vi "DuelistTactic.vi"(9 "Game in":refnum<class "Game.lvclass">, 10 "Robot":refnum<class "Robot.lvclass">, 11 "DuelistTactic in":refnum<class "DuelistTactic.lvclass">) -> (2 "Robot out":refnum<class "Robot.lvclass">, 3 "DuelistTactic out":refnum<class "DuelistTactic.lvclass">)   [LabVIEW 2020, in "DuelistTactic.lvclass"]
uses:
  DuelistTactic.lvclass
  C:/Users/anton/Desktop/RoboIME/IC/SSL_AI/Tactic_class/Tactic.lvclass
  Robot_class/Robot.lvclass
  Game_class/Game.lvclass
  Robot_class/tactics.ctl
  Tactic_class/Tactic.lvclass/Tactic.ctl
  Robot_class/Robot.lvclass/Robot.ctl
  Tactic_class/Read Skillbook.vi
  Robot_class/Write tactic.vi
  Skillbook_class/Skillbook.lvclass
  DuelistSkill_class/DuelistSkill.lvclass
panel:
  out "x .or. y?":bool
  out "error out 2":errorcluster
  in  "error in (no error) 2":errorcluster
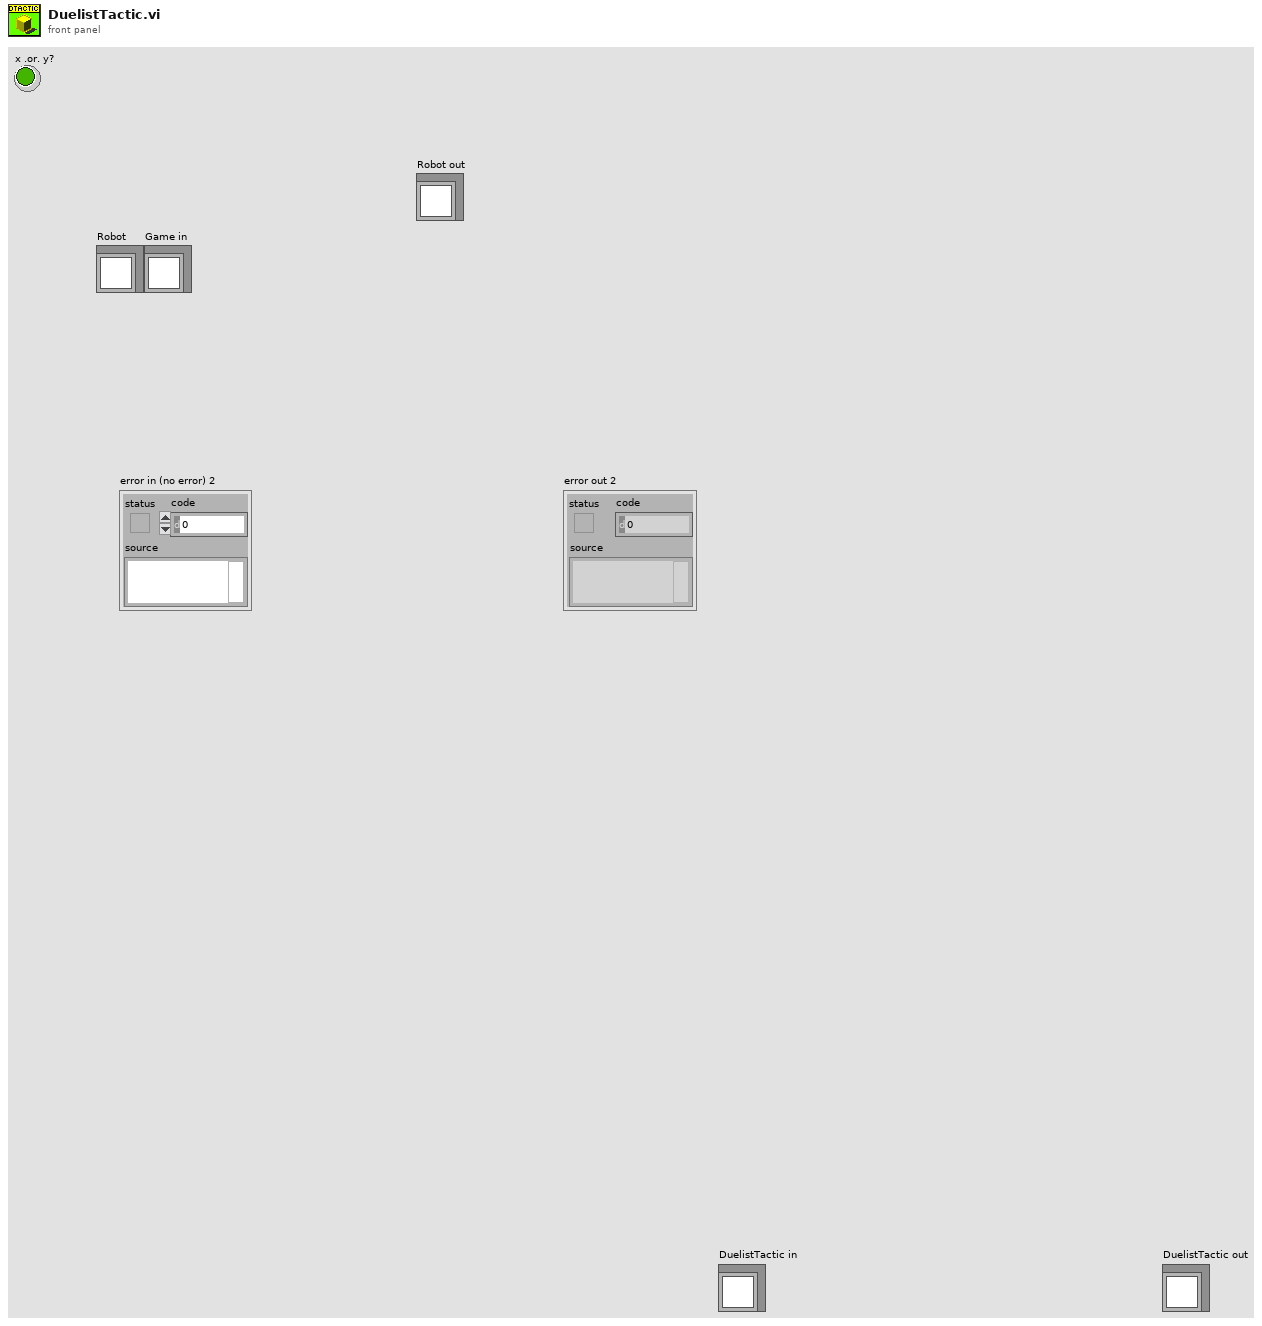
[diagram p1: front panel]
types:
  T1 = typedef "tactics.ctl" = enum16{"GoToBallPlacementPosition", "PlaceBall", "GoToBallPlacement", "5Robots", "BallPlacementEnemy", "ReceivePassInFuturePoint", "Roller", "PrepareRollToPassRollerGoTo", "PrepareRollToPassReceiverGoTo", "WaitRoll", "PositionToRoll", "PenaltyAttacker", "PassObserver", "PenaltyDefense", "TableReceiverTactic", "Test", "DefendGoal", "Marker", "FollowAttacker", "DefendArea", "Shoot", "AttackerAimGoal", "AttackerBallOutOfField", "AttackerBlock", "AttackerStop", "Duelist", "Halt", "ZigZag", "GoTo", "Timeout", "KickToBestRobot", "KickToPassReceiver", "PositionToReceivePass", "WaitPass"}
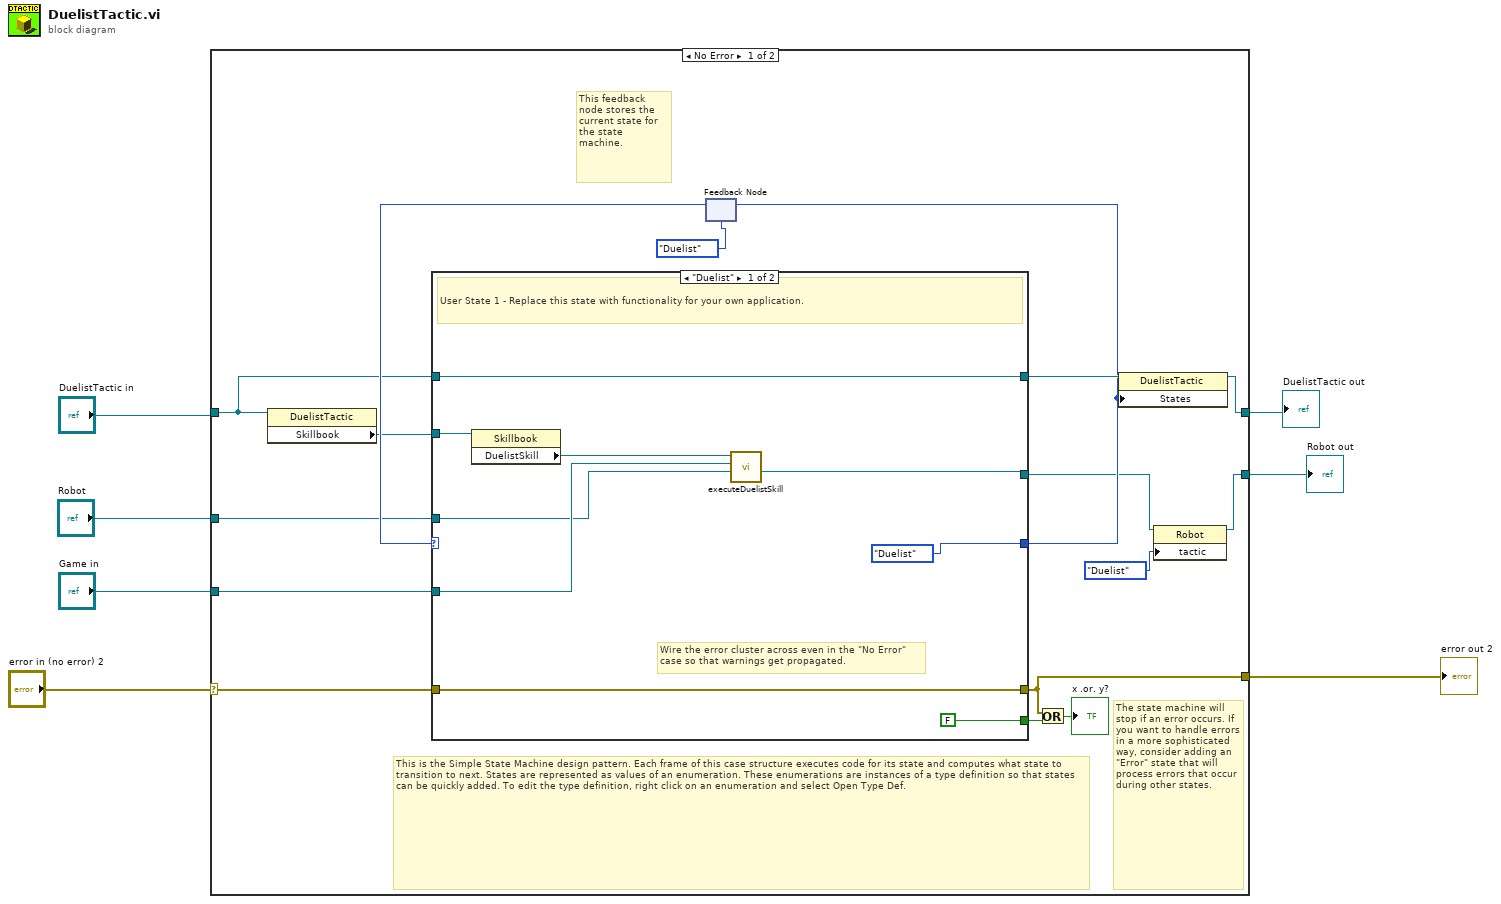
[diagram p0: block diagram]
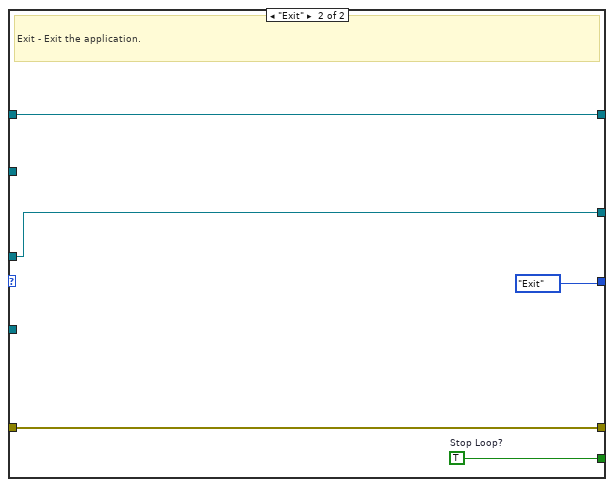
[diagram p2: hidden frame]
diagram:
  n1 = case shown="No Error" "error in (no error) 2" {
    selector: "error in (no error) 2" -> [w20 w40]
    tunnel: [w19 w40] -> w6
    tunnel: [w14 w39] -> w1
    tunnel: "DuelistTactic in" -> [w17 w39]
    tunnel: "Robot" -> [w18 w38]
    tunnel: [w8 w38] -> w4
    tunnel: "Game in" -> [w12 _]
    frame No Error {
      # "The state machine will stop if an error occurs. If you want to handle errors in a more sophisticated way, consider adding an \"Error\" state that will process errors that occur during other states."
      # "This feedback node stores the current state for the state machine."
      # "This is the Simple State Machine design pattern. Each frame of this case structure executes code for its state and computes what state to transition to next. States are represented as values of an enumeration. These enumerations are instances of a type definition so that states can be quickly added. To edit the type definition, right click on an enumeration and select Open Type Def."
      # "Wire the error cluster across even in the \"No Error\"\ncase so that warnings get propagated."
      n2 = property class="DuelistTactic"(reference=w17) -> ("Skillbook"=w16:refnum<class "Skillbook.lvclass">)  [unwired: 1 in, 2 out]
      n3 = feedback #1(enum16{"Duelist", "Exit"}."Duelist" ("y")) -> (w21:enum16{"Duelist", "Exit"})
      n4 = case shown="\"Duelist\"" w21 {
        tunnel: [enum16{"Duelist", "Exit"}."Duelist" ("y") enum16{"Duelist", "Exit"}."Exit" ("y")] -> w13
        tunnel: [FALSE ("Stop Loop?") w37] -> w23
        tunnel: w20 -> [w31 w36]
        tunnel: [w31 w36] -> w19
        tunnel: w16 -> [w30 _]
        tunnel: w18 -> [w25 w35]
        tunnel: [w24 w35] -> w9
        tunnel: [w29 w34] -> w15
        tunnel: w17 -> [w29 w34]
        tunnel: w12 -> [w27 _]
        frame "Duelist" {
          # "User State 1 - Replace this state with functionality for your own application."
          n5 = property class="Skillbook"(reference=w30) -> ("DuelistSkill"=w28:refnum<class "DuelistSkill.lvclass">)  [unwired: 1 in, 2 out]
          n6 = call "executeDuelistSkill.vi"("Duelist Robot in"=w25, "Game"=w27, "DuelistSkill in"=w28) -> ("Duelist Robot out"=w24:refnum<class "Robot.lvclass">)  [unwired: 6 in, 2 out]
        }
        frame "Exit" {
          w37 = TRUE  # Stop Loop?
          # "Exit - Exit the application."
        }
      }
      n7 = feedback-in #1(w13) -> ()
      n8 = Or(x=w19, y=w23) -> (x .or. y?=→"x .or. y?":bool)
      n9 = property class="DuelistTactic"(reference=w15, "States"=w13) -> (reference out=w14:refnum<class "DuelistTactic.lvclass">)  [unwired: 1 in, 1 out]
      n10 = property class="Robot"(reference=w9, "tactic"=tactics."Duelist") -> (reference out=w8:refnum<class "Robot.lvclass">)  [unwired: 1 in, 1 out]
    }
    frame Error {
    }
  }
  "DuelistTactic out" <- w1
  "error out 2" <- w6
  "Robot out" <- w4
